vi "spliteFTPpathLeaf.vi"(11 "Name":string) -> (3 "String":string)   [LabVIEW 2014]
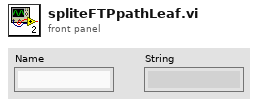
[diagram p1: front panel]
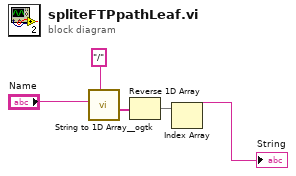
[diagram p0: block diagram]
diagram:
  n1 = call <userlib>:"String to 1D Array__ogtk.vi"("delimiter (Tab)"="/", "string"="Name") -> ("Array of Strings"=w4:string[])  [unwired: 9 in]
  n2 = Reverse 1D Array(array=w4) -> (reversed array=w3:string[])
  n3 = Index Array(array=w3) -> (element=→"String":string)  [unwired: 1 in]
